vi "Pockels Cal-Default percentage to volts convertion.vi"(11 "Pockels power":dbl) -> (3 "Pockels Volts":dbl)   [LabVIEW 2013]
uses:
  <vilib>/gmath/NI_Gmath.lvlib
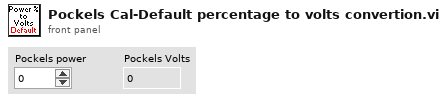
[diagram p1: front panel]
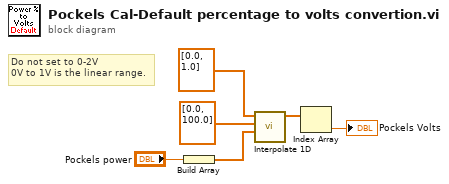
[diagram p0: block diagram]
diagram:
  # "Do not set to 0-2V\n0V to 1V is the linear range."
  n1 = Build Array("Pockels power") -> (w4:dbl[])
  n2 = call <vilib>:"Interpolate 1D.vi"("xi"=w4, "X"=dbl[] [0.0, 100.0] ("Y"), "Y"=dbl[] [0.0, 1.0]) -> ("yi"=w5:dbl[])  [unwired: 6 in, 2 out]
  n3 = Index Array(array=w5) -> (element=→"Pockels Volts":dbl)  [unwired: 1 in]
